vi "Tryk_Måler_SUBVI.vi"(10 "element":dbl[](array[numeric]), 11 "Array in":dbl[](array[numeric])) -> (2 "Tryk_Hoej":dbl[](array[numeric]), 3 "Tryk_Lav":dbl[](array[numeric]))   [LabVIEW 2022 SP3]
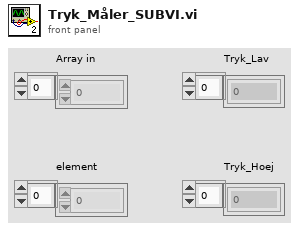
[diagram p1: front panel]
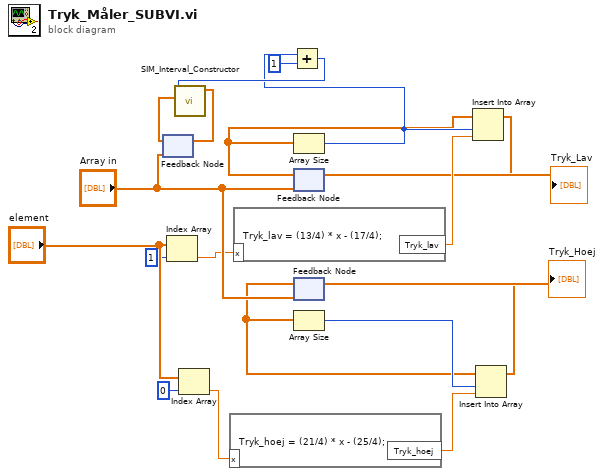
[diagram p0: block diagram]
diagram:
  n1 = feedback #1("Array in") -> (w5:dbl[])
  n2 = Index Array(array="element", index=1) -> (element=w4:dbl)
  n3 = Index Array(array="element", index=0) -> (element=w3:dbl)
  n4 = formula code="Tryk_hoej = (21/4) * x - (25/4);"("x"=w3) -> ("Tryk_hoej"=w13:dbl)
  n5 = formula code="Tryk_lav = (13/4) * x - (17/4);"("x"=w4) -> ("Tryk_lav"=w9:dbl)
  n6 = feedback #2("Array in") -> (w8:dbl[])
  "Tryk_Lav" <- w8
  n7 = Array Size(array=w8) -> (size(s)=w15:i32)
  n8 = Add(x=w15, y=1) -> (x+y=w17:i32)
  n9 = call "SIM_Interval_Constructor.vi"("History Data in"=w5, "size(s)"=w17) -> ("History Data out"=w6:dbl[])  [unwired: 9 in]
  n10 = feedback-in #1(w6) -> ()
  n11 = feedback #3("Array in") -> (w11:dbl[])
  "Tryk_Hoej" <- w11
  n12 = Array Size(array=w11) -> (size(s)=w12:i32)
  n13 = Insert Into Array(array=w8, index=w15, new element=w9) -> (w7:dbl[])
  n14 = feedback-in #2(w7) -> ()
  n15 = Insert Into Array(array=w11, index=w12, new element=w13) -> (w10:dbl[])
  n16 = feedback-in #3(w10) -> ()
